vi "State_Machine.vi"(8 "error in (no error)":errorcluster caption="entrée d'erreur (pas d'erreur)", 11 "Get_Voltage en entrée":refnum<class "Show_Result_Relay.lvclass">) -> (0 "error out":errorcluster caption="sortie d'erreur", 2 "Json_String":string, 3 "Get_Voltage en sortie":refnum<class "Show_Result_Relay.lvclass">)   [LabVIEW 2020, in "Library Test.lvlib" / "Show_Result_Relay.lvclass"]
uses:
  Show_Result_Relay.lvclass
  C:/Users/ngarcin/OneDrive - Altyor/Standard TB/Suite TB45/Class/Test/Test (Default)/Test (Default).lvclass
  Commun VI/TypeDef/Commande Relay_Board/Parameter Relay_Board.ctl
  Relay_Board/Relay_Board (Default)/Class Relay_Board (Default).lvclass
  Commun VI/TypeDef/Variable Printable.ctl
  Commun VI/TypeDef/Commande Relay_Board/Data_Write_Relay_Board.ctl
  Show_Result_Relay.lvclass/Show_Result_Relay.ctl
  JSON API/JSON Value/Set from JSON string.vi
  JSON API/Variant JSON/Variant to JSON.vi
  JSON API/JSON Value/Get Item by name array.vi
  Instrument/Instrument (Default)/Class Instrument (Default).lvclass
  JSON API/JSON Value/JSON Value.lvclass
  Commun VI/Library Commun.lvlib
  JSON API/Variant JSON/Variant JSON.lvlib
  JSON API/Get Polymorphic/JSON GetSet.lvlib
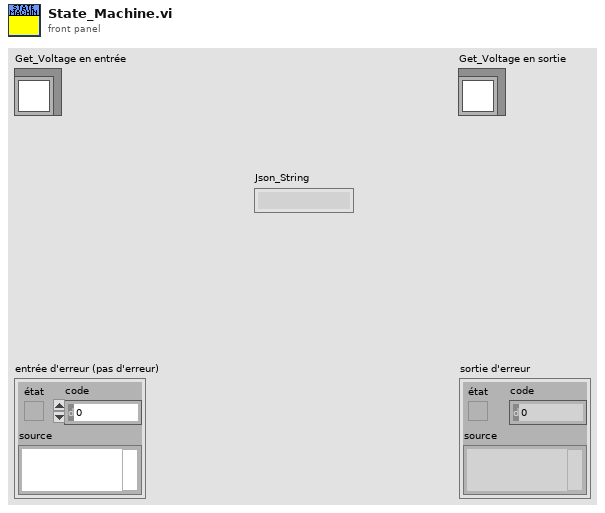
[diagram p1: front panel]
types:
  T1 = typedef "Library Commun.lvlib/Data_Write_Relay_Board.ctl" = enum16{"Enable Relays", "Disable Relays"}
  T2 = typedef "Variable Printable.ctl" = string
  T3 = enum16{"Get Variable", "Get All Variables", "Set Variable", "Delete Variable", "Delete All Variable"}
  T4 = typedef "Library Commun.lvlib/Parameter Relay_Board.ctl" = cluster{"Device_Com_Port":string, "Address Board":string, "Tab_Num_Relay":u8[], "Parameter Class Relay_Board":refnum<class "Class Relay_Board (Default).lvclass">}
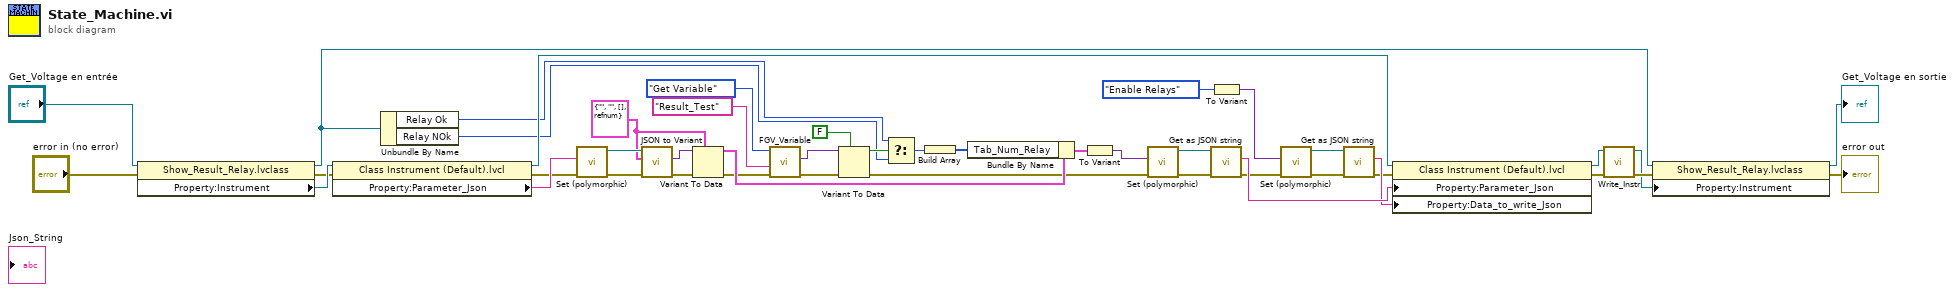
[diagram p0: block diagram]
diagram:
  w36 = T4 {"Device_Com_Port"="", "Address Board"="", "Tab_Num_Relay"=[], "Parameter Class Relay_Board"=refnum} ("Parameter")
  n1 = property class="Show_Result_Relay.lvclass"(reference="Get_Voltage en entrée", error in="error in (no error)") -> (reference out=w17:refnum<class "Show_Result_Relay.lvclass">, error out=w23:errorcluster, "Property:Instrument"=w24:refnum<class "Class Instrument (Default).lvclass">)
  n2 = property class="Class Instrument (Default).lvcl"(reference=w24, error in=w23) -> (reference out=w44:refnum<class "Class Instrument (Default).lvclass">, error out=w38:errorcluster, "Property:Parameter_Json"=w39:string)
  n3 = Unbundle By Name(w17) -> ("Relay Ok"=w15:i32, "Relay NOk"=w14:i32)
  n4 = call-poly "Set (polymorphic).vi"("error in (no error)"=w38, "JSON stream"=w39) -> ("error out"=w41:errorcluster, "JSON Value out"=w43:refnum<class "JSON Value.lvclass">)  [unwired: 7 in, 1 out]
  n5 = call "JSON to Variant.vi"("error in (no error)"=w41, "Variant (Data Type)"=w36, "JSON Value"=w43) -> ("error out"=w42:errorcluster, "Variant out"=w40:variant)  [unwired: 7 in]
  n6 = Variant To Data(error in=w42, type=w36, Variant=w40) -> (data=w37:T4, error out=w19:errorcluster)
  n7 = call "FGV_Variable.vi"("error in (no error)"=w19, "Variable"=T2 "Result_Test", "Function"=T3."Get Variable") -> ("error out"=w28:errorcluster, "Data Out"=w27:variant)  [unwired: 6 in, 1 out]
  n8 = Variant To Data(error in=w28, type=FALSE, Variant=w27) -> (data=w16:bool, error out=w18:errorcluster)
  n9 = Select(t=w15, s=w16, f=w14) -> (s? t:f=w13:i32)
  n10 = Build Array(w13) -> (w12:i32[])
  n11 = Bundle By Name(cluster=w37, "Tab_Num_Relay"=w12) -> (w34:T4)
  n12 = To Variant(anything=w34) -> (Variant=w33:variant)
  n13 = call-poly "Set (polymorphic).vi"("error in (no error)"=w18, "Variant"=w33) -> ("error out"=w31:errorcluster, "JSON Value out"=w35:refnum<class "JSON Value.lvclass">)  [unwired: 8 in]
  n14 = call "Get as JSON string.vi"("error in (no error)"=w31, "JSON Value in"=w35) -> ("error out"=w2:errorcluster, "<JSON>"=w32:string)  [unwired: 8 in]
  n15 = To Variant(anything=Data_Write_Relay_Board."Enable Relays" ("Function")) -> (Variant=w11:variant)
  n16 = call-poly "Set (polymorphic).vi"("error in (no error)"=w2, "Variant"=w11) -> ("error out"=w10:errorcluster, "JSON Value out"=w3:refnum<class "JSON Value.lvclass">)  [unwired: 8 in]
  n17 = call "Get as JSON string.vi"("error in (no error)"=w10, "JSON Value in"=w3) -> ("error out"=w1:errorcluster, "<JSON>"=w4:string)  [unwired: 8 in]
  n18 = property class="Class Instrument (Default).lvcl"(reference=w44, error in=w1, "Property:Parameter_Json"=w32, "Property:Data_to_write_Json"=w4) -> (reference out=w8:refnum<class "Class Instrument (Default).lvclass">, error out=w5:errorcluster)
  n19 = call-dynamic "Write_Instr.vi"("error in (no error)"=w5, "Class Multimeter (Default) en entrée"=w8) -> ("error out"=w7:errorcluster, "Class Multimeter (Default) en sortie"=w6:refnum<class "Class Instrument (Default).lvclass">)  [unwired: 8 in]
  n20 = property class="Show_Result_Relay.lvclass"(reference=w17, error in=w7, "Property:Instrument"=w6) -> (reference out=→"Get_Voltage en sortie":refnum<class "Show_Result_Relay.lvclass">, error out=→"error out":errorcluster)
